vi "acq.saveIntermediary.vi"(5 "camera in":refnum<class "camera.lvclass">, 7 "name":string, 8 "error in":errorcluster, 10 "acq.# Acq":u16, 11 "path":path) -> (0 "error out":errorcluster)   [LabVIEW 2020]
uses:
  camera/camera.lvclass
  _controls/imageType.ctl
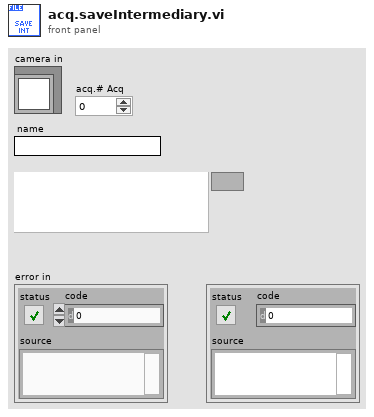
[diagram p1: front panel]
types:
  T1 = typedef "imageType.ctl" = enum16{"dark", "bright"}
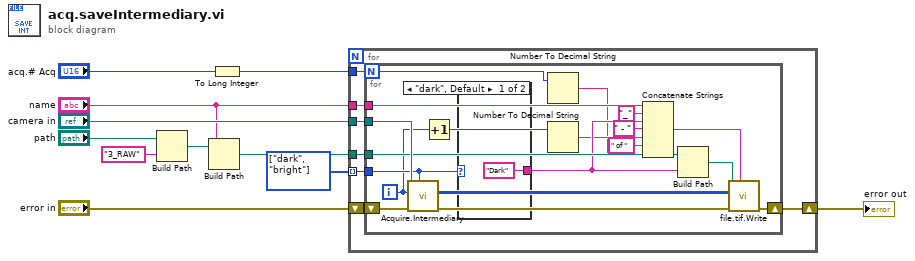
[diagram p0: block diagram]
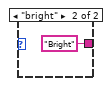
[diagram p2: hidden frame]
diagram:
  w9 = T1[] [enum."dark", enum."bright"] items=["dark", "bright"] ("type")
  n1 = Build Path(base path="path", name or relative path="3_RAW") -> (appended path=w6:path)
  n2 = Build Path(base path=w6, name or relative path="name") -> (appended path=w4:path)
  n3 = To Long Integer(number="acq.# Acq") -> (32bit integer=w1:i32)
  n4 = for {
    tunnel: "camera in" -> [w17]
    tunnel: w9 -> [w16] mode=indexing
    shift-right: [w15] -> w8
    shift-left: "error in" -> [w18]
    tunnel: w4 -> [w14]
    tunnel: "name" -> [w13]
    tunnel: w1 -> [w12]
    n5 = for {
      N: w12 -> [w22]
      tunnel: w17 -> [w34]
      tunnel: w16 -> [w32]
      shift-right: [w35] -> w15
      shift-left: w18 -> [w37]
      tunnel: w14 -> [w31]
      tunnel: w13 -> [w29]
      i -> [w25]
      n6 = call-dynamic "Acquire.Intermediary.vi"("type"=w32, "error in"=w37, "index"=w25, "camera.nit in"=w34) -> ("error out"=w36:errorcluster, "buffer"=w33:u16[][])  [unwired: 6 in]
      n7 = Increment(x=w25) -> (x+1=w19:i32)
      n8 = case shown="\"dark\", Default" w32 {
        tunnel: ["Dark" "Bright"] -> w27
        frame "dark", Default {
        }
        frame "bright" {
        }
      }
      n9 = Number To Decimal String(number=w22) -> (decimal integer string=w21:string)  [unwired: 1 in]
      n10 = Number To Decimal String(number=w19) -> (decimal integer string=w24:string)  [unwired: 1 in]
      n11 = Concatenate Strings(w29, "_" ("string"), w27, " - " ("string"), w24, " of " ("string"), w21) -> (w26:string)
      n12 = Build Path(base path=w31, name or relative path=w27) -> (appended path=w30:path)
      n13 = call "file.tif.Write.vi"("name"=w26, "error in"=w36, "u16 pixmap"=w33, "path"=w30) -> ("error out"=w35:errorcluster)  [unwired: 7 in]
    }
  }
  "error out" <- w8
